vi "laserpid.vi"(0 "TCP Array":refnum<k5>[](array[refnum]), 1 "Set wave Array":dbl[](array[numeric]) format="%.6f", 2 "Lock Array":bool[](array[boolean]), 3 "Numeric":i16, 4 "Set volt Array 0":dbl[](array[numeric]) format="%.6f", 5 "waring in":bool, 7 "PID gains":T1={"proportional gain (Kc)"=1000.0, "integral time (Ti, min)"=0.0, "derivative time (Td, min)"=0.0} {"derivative time (Td, min)" format="%.3f"; "integral time (Ti, min)" format="%.3f"; "proportional gain (Kc)" format="%.3f"}) -> (6 "warning out":bool, 8 "wavelenth":string)   [LabVIEW 2014]
uses:
  <vilib>/addons/control/pid/pid.llb/PID (DBL).vi
  <vilib>/addons/control/pid/NI_PID_pid.lvlib
  wlmData.dll
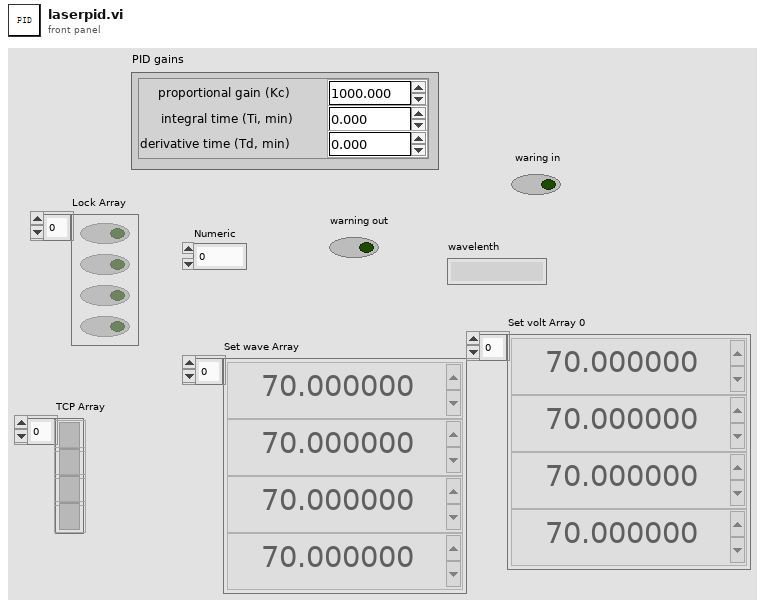
[diagram p1: front panel]
types:
  T1 = cluster{"proportional gain (Kc)":dbl, "integral time (Ti, min)":dbl, "derivative time (Td, min)":dbl}
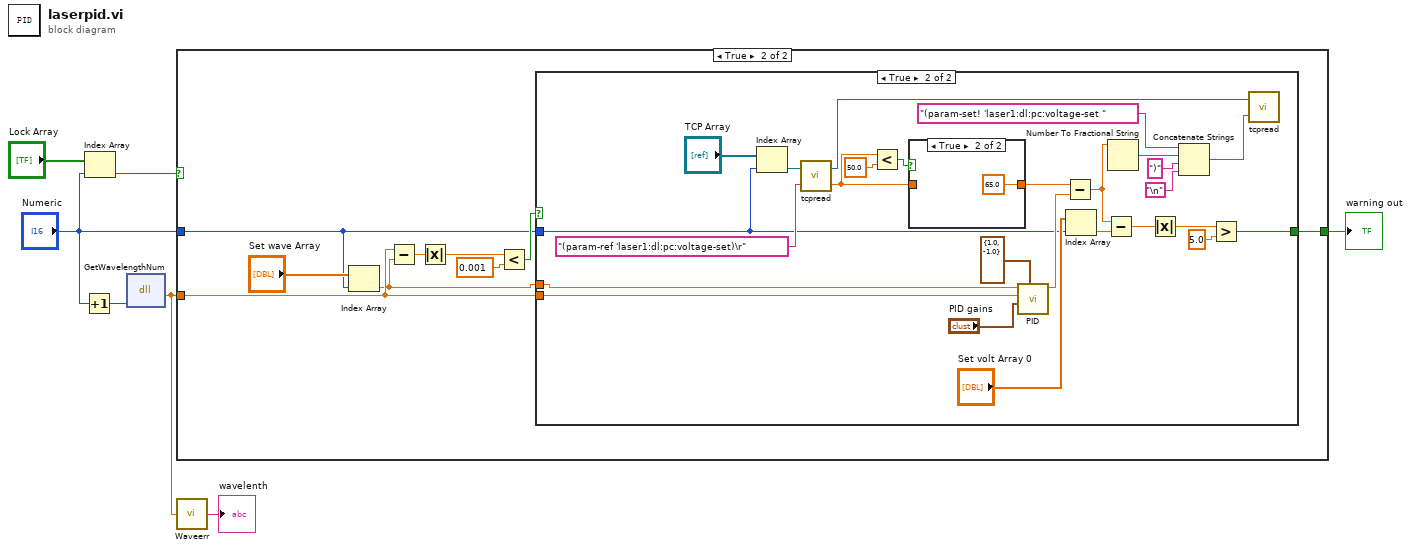
[diagram p0: block diagram]
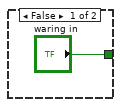
[diagram p2: hidden frame]
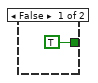
[diagram p3: hidden frame]
diagram:
  n1 = Increment(x="Numeric") -> (x+1=w4:i16)
  n2 = Index Array(array="Lock Array", index="Numeric") -> (element=w6:bool)
  n3 = dll-call lib="wlmData.dll" fn="GetWavelengthNum"("channel"=w4) -> ("res"=w1:dbl)  [unwired: 4 in, 2 out]
  n4 = case shown="True" w6 {
    tunnel: "Numeric" -> [_ w10]
    tunnel: ["waring in" w17] -> w2
    tunnel: w1 -> [_ w12]
    frame False {
    }
    frame True {
      n5 = Index Array(array="Set wave Array", index=w10) -> (element=w9:dbl)
      n6 = Subtract(x=w12, y=w9) -> (x-y=w14:dbl)
      n7 = Absolute Value(x=w14) -> (abs(x)=w16:dbl)
      n8 = Less?(x=w16, y=0.001) -> (x < y?=w13:bool)
      n9 = case shown="True" w13 {
        tunnel: w10 -> [_ w31]
        tunnel: [TRUE w26] -> w17
        tunnel: w12 -> [_ w24]
        tunnel: w9 -> [_ w23]
        frame False {
        }
        frame True {
          n10 = Index Array(array="TCP Array", index=w31) -> (element=w33:refnum<k5>)
          n11 = call "tcpread.vi"("String 2"="(param-ref 'laser1:dl:pc:voltage-set)\r" ("write buffer"), "TCP Network Connection Refnum"=w33) -> ("OUT"=w20:dbl, "TCP Network Connection Refnum 2"=w35:refnum<k5>)
          n12 = Less?(x=w20, y=50.0) -> (x < y?=w21:bool)
          n13 = case shown="True" w21 {
            tunnel: [w45 65.0] -> w19
            tunnel: w20 -> [w45 _]
            frame False {
            }
            frame True {
            }
          }
          n14 = call-poly <vilib>:"PID.vi"("output range"=cluster{"output high":dbl, "output low":dbl} {"output high"=1.0, "output low"=-1.0}, "PID gains"="PID gains", "process variable"=w24, "setpoint"=w23) -> ("output"=w44:dbl)  [unwired: 6 in, 1 out]
          n15 = Subtract(x=w19, y=w44) -> (x-y=w30:dbl)
          n16 = Index Array(array="Set volt Array 0", index=w31) -> (element=w25:dbl)
          n17 = Subtract(x=w30, y=w25) -> (x-y=w29:dbl)
          n18 = Number To Fractional String(number=w30) -> (F-format string=w38:string)  [unwired: 3 in]
          n19 = Absolute Value(x=w29) -> (abs(x)=w28:dbl)
          n20 = Concatenate Strings("(param-set! 'laser1:dl:pc:voltage-set " ("string"), w38, ")" ("string"), "\n") -> (w41:string)
          n21 = Greater?(x=w28, y=5.0) -> (0:w26:bool)
          n22 = call "tcpread.vi"("String 2"=w41, "TCP Network Connection Refnum"=w35) -> ()  [unwired: 2 out]
        }
      }
    }
  }
  "warning out" <- w2
  n23 = call "Waveerr.vi"("Numeric"=w1) -> ("String"=→"wavelenth":string)
